vi "FormatLimitAction.vi"(1 "Limit action":T1) -> (0 "value":string)   [LabVIEW 2014, in "Raspberry Pi Compatible Compiler for LabVIEW.lvlib" / "PythonConfiguration.lvclass"]
uses:
  PythonConfiguration.lvclass
  TypeDefs/LimitAction.ctl
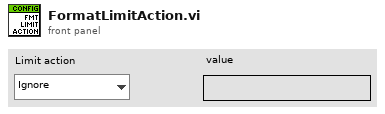
[diagram p1: front panel]
types:
  T1 = typedef "Raspberry Pi Compatible Compiler for LabVIEW.lvlib/PythonConfiguration.lvclass/LimitAction.ctl" = enum8{"Ignore", "Coerce"}
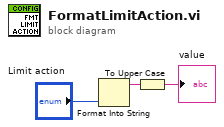
[diagram p0: block diagram]
diagram:
  n1 = Format Into String("Limit action") -> (resulting string=w2:string)  [unwired: 3 in, 1 out]
  n2 = To Upper Case(1:w2) -> (0:→"value":string)
